vi "CopyImage.vi"(1 "DST":T1(plugin-control)=refnum, 2 "SRC":T1(plugin-control)=refnum) -> (0 "Image out":T1(plugin-control))   [LabVIEW 2015]
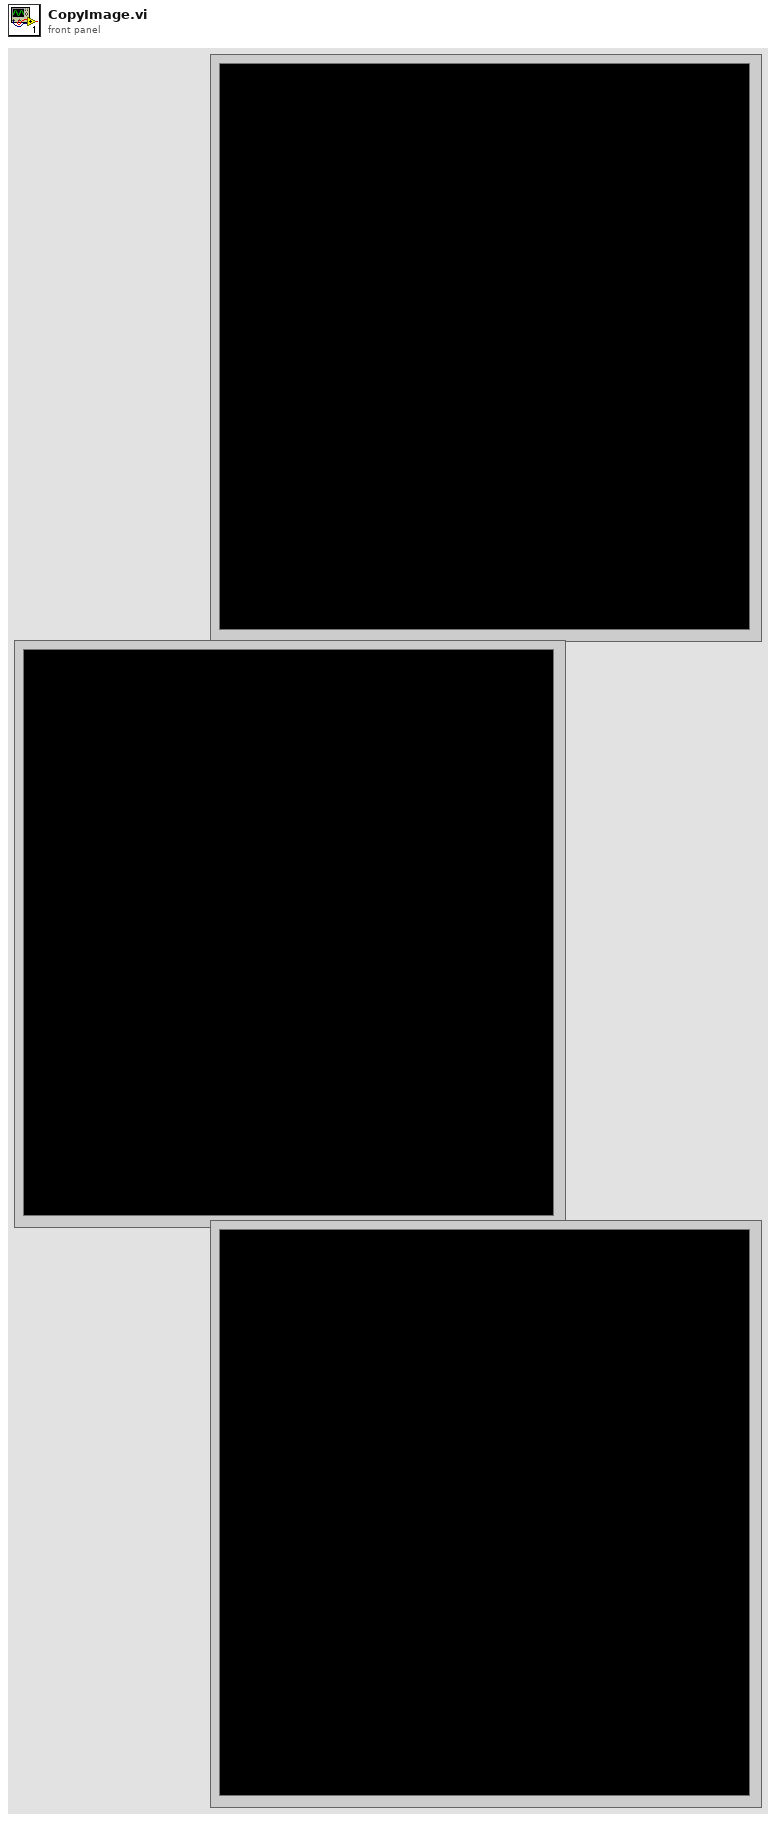
[diagram p1: front panel]
types:
  T1 = typedef "IMAQ Image.ctl" = refnum<image>
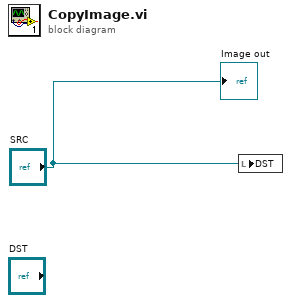
[diagram p0: block diagram]
diagram:
  n1 = local write "DST"("SRC") -> ()
  "Image out" <- "SRC"
